vi "Panel Create.vi"(10 "Panel":refnum<class "Panel.lvclass">, 11 "Panel Create in":refnum<class "Panel Create.lvclass">) -> (3 "Panel Create out":refnum<class "Panel Create.lvclass">)   [LabVIEW 2021, in "Panel Create.lvlib" / "Panel Create.lvclass"]
uses:
  Panel Create.lvclass
  Panel/Panel.lvclass
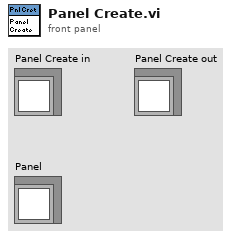
[diagram p1: front panel]
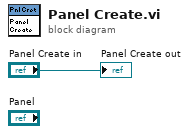
[diagram p0: block diagram]
diagram:
  "Panel Create out" <- "Panel Create in"
